vi "Get Channel Identifiers.vi"(8 "error in":errorcluster, 11 "Thermometer Multichannel in":refnum<class "Thermometer Multichannel.lvclass">) -> (0 "error out":errorcluster, 2 "Channel Identifiers":string[](array[string]), 3 "Thermometer Multichannel out":refnum<class "Thermometer Multichannel.lvclass">)   [LabVIEW 2024, in "Thermometer Multichannel.lvclass"]
uses:
  Thermometer Multichannel.lvclass
  Interfaces/IRead Temperature Multichannel/IRead Temperature Multichannel.lvclass
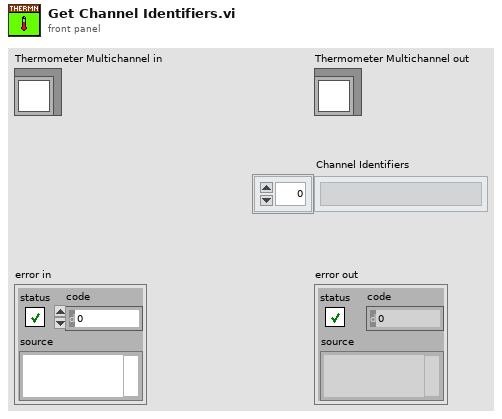
[diagram p1: front panel]
types:
  T1 = typedef "Thermometer Multichannel.lvclass/ObjectAttributes.ctl" = cluster{"IConfigure":refnum<class "IConfigure.lvclass">, "Worker Enqueuer":refnum<class "Message Enqueuer.lvclass">}
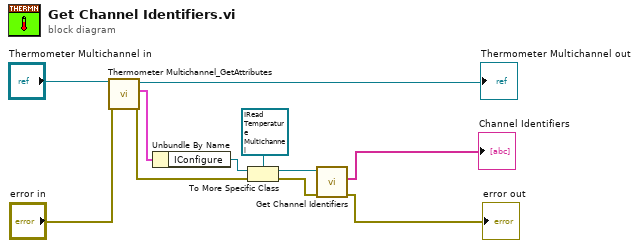
[diagram p0: block diagram]
diagram:
  n1 = call "Thermometer Multichannel_GetAttributes.vi"("Error In"="error in", "reference in"="Thermometer Multichannel in") -> ("Error Out"=w6:errorcluster, "Data"=w9:T1, "reference out"=→"Thermometer Multichannel out":refnum<class "Thermometer Multichannel.lvclass">)  [unwired: 6 in, 1 out]
  n2 = Unbundle By Name(w9) -> ("IConfigure"=w8:refnum<class "IConfigure.lvclass">)
  n3 = To More Specific Class(target class=refnum<class "IRead Temperature Multichannel.lvclass"> refnum ("IRead Temperature Multichannel.lvclass"), reference=w8, error in=w6) -> (specific class reference=w5:refnum<class "IRead Temperature Multichannel.lvclass">, error out=w4:errorcluster)
  n4 = call-dynamic "Get Channel Identifiers.vi"("error in"=w4, "IRead Temperature Multichannel in"=w5) -> ("error out"=→"error out":errorcluster, "Channel Identifiers"=→"Channel Identifiers":string[])  [unwired: 7 in, 1 out]
